vi "SVT Unit Conversion (1 Ch).vi"(0 "spectrum":cluster{"x0":dbl, "dx":dbl, "magnitude":dbl[]} {"magnitude" format="%.2p"; "dx" format="%.2p"; "x0" format="%.2p"}, 1 "desired scaling":T2 {"dB reference (0: no change)" format="%.2f"}, 2 "spectral density desired":T1(ring), 4 "spectrum info in":T3={"channel name"="", "description"="", "x-axis units"=0, "spectral info"={"spectrum type"=enum."Power [Magnitude^2]", "linear/dB"=enum."linear", "window"=0, "window size"=0, "FFT size"=0}, "engineering units"=0, "custom label"="", "dB reference [EU]"=0.0, "peak units"=enum."rms", "weighting filter"=0, "spectral density?"=FALSE, "unit label"="", "spectrum skewed?"=FALSE, "complimentary spectrum units"=enum."none"} {"x-axis units" items=["time"=0, "frequency"=1, "quefrency"=2, "revolutions"=3, "order"=4, "rpm"=11, "rad/s"=21, "index"=65535]; "weighting filter" items=["Linear", "A-weighting", "B-weighting", "C-weighting", "ITU-R 468-4", "Dolby", "CCITT", "C-message"]; "dB reference [EU]" format="%.2f"; "engineering units" items=["custom..."=0, "V"=1, "A"=21, "Pa"=2, "N"=20, "g"=3, "m/s^2"=4, "m/s"=5, "m"=6, "mm/s"=12, "mm"=13, "microns/s"=14, "microns"=15, "in/s^2"=7, "in/s"=8, "in"=9, "mils/s"=10, "mils"=11, "rad/s^2"=16, "rad/s"=17, "rad"=18, "strain"=19]; "spectral info"."window" items=["None "=0, "Hanning"=1, "Hamming"=2, "Blackman-Harris"=3, "Exact Blackman"=4, "Blackman"=5, "Flat Top"=6, "4 Term B-Harris "=7, "7 Term B-Harris"=8, "Low Sidelobe"=9, "Force - Exponential"=10, "Gaussian"=62]}, 5 "error in (no error)":errorcluster) -> (14 "converted spectrum":cluster{"x0":dbl, "dx":dbl, "magnitude":dbl[]} {"magnitude" format="%.2p"; "dx" format="%.2p"; "x0" format="%.2p"}, 15 "unit label":string, 18 "spectrum info out":T3={"channel name"="", "description"="", "x-axis units"=0, "spectral info"={"spectrum type"=enum."Power [Magnitude^2]", "linear/dB"=enum."linear", "window"=0, "window size"=0, "FFT size"=0}, "engineering units"=0, "custom label"="", "dB reference [EU]"=0.0, "peak units"=enum."rms", "weighting filter"=0, "spectral density?"=FALSE, "unit label"="", "spectrum skewed?"=FALSE, "complimentary spectrum units"=enum."none"} {"x-axis units" items=["time"=0, "frequency"=1, "quefrency"=2, "revolutions"=3, "order"=4, "rpm"=11, "rad/s"=21, "index"=65535]; "weighting filter" items=["Linear", "A-weighting", "B-weighting", "C-weighting", "ITU-R 468-4", "Dolby", "CCITT", "C-message"]; "dB reference [EU]" format="%.2f"; "engineering units" items=["custom..."=0, "V"=1, "A"=21, "Pa"=2, "N"=20, "g"=3, "m/s^2"=4, "m/s"=5, "m"=6, "mm/s"=12, "mm"=13, "microns/s"=14, "microns"=15, "in/s^2"=7, "in/s"=8, "in"=9, "mils/s"=10, "mils"=11, "rad/s^2"=16, "rad/s"=17, "rad"=18, "strain"=19]; "spectral info"."window" items=["None "=0, "Hanning"=1, "Hamming"=2, "Blackman-Harris"=3, "Exact Blackman"=4, "Blackman"=5, "Flat Top"=6, "4 Term B-Harris "=7, "7 Term B-Harris"=8, "Low Sidelobe"=9, "Force - Exponential"=10, "Gaussian"=62]}, 19 "error out":errorcluster)   [LabVIEW 2017]
doc: "Converts between dB/linear, Magnitude/Magnitude^2, rms/peak/peak-peak, spectrum/spectral density, and dB ref1/dB ref2. You can use this polymorphic VI to convert a single spectrum, N spectra, a single complex spectrum, N complex spectra, a single channel of XY data, or N channels of XY data. The data type you wire to the <B>spectrum</B> input determines the polymorphic instance to use."
uses:
  <vilib>/addons/Sound and Vibration/compatibility/Controls/svl_Spectrum Info (enhanced).ctl
  <vilib>/addons/Sound and Vibration/compatibility/Controls/svl_Spectrum Type.ctl
  <vilib>/addons/Sound and Vibration/compatibility/Controls/svl_Engineering Units Text Ring.ctl
  <vilib>/addons/Sound and Vibration/compatibility/Controls/svl_Weighting Filter Text Ring.ctl
  <vilib>/addons/Sound and Vibration/compatibility/Controls/svl_Complimentary Spectrum Units.ctl
  <vilib>/addons/_NISVFA/_Spectrum Processing/subVIs/svfa_Peak to RMS to Peak2Peak.vi
  <vilib>/addons/_NISVFA/_Spectrum Processing/subVIs/svfa_Mag to Mag2.vi
  <vilib>/addons/_NISVFA/_Spectrum Processing/subVIs/svfa_Linear to dB.vi
  <vilib>/addons/_NISVFA/_Spectrum Processing/subVIs/svfa_dBrefA to dBrefB.vi
  <vilib>/addons/_NISVFA/_Spectrum Processing/subVIs/svfa_Spectrum to Spectral Density.vi
  <vilib>/addons/_NISVFA/_Shared subVIs/Common/svc_Get Weighting Enum and Labels.vi
  <vilib>/addons/_NISVFA/_Shared subVIs/Common/svc_Unit Label Lexical Class.vi
  <vilib>/addons/_NISVFA/_Shared subVIs/Common/svc_Engineering Units to Unit Label.vi
  <vilib>/addons/_NISVFA/_Shared subVIs/Common/svc_Format Value (DBL).vi
  <vilib>/addons/_NISVFA/_Shared subVIs/Common/svc_Window Parameters.vi
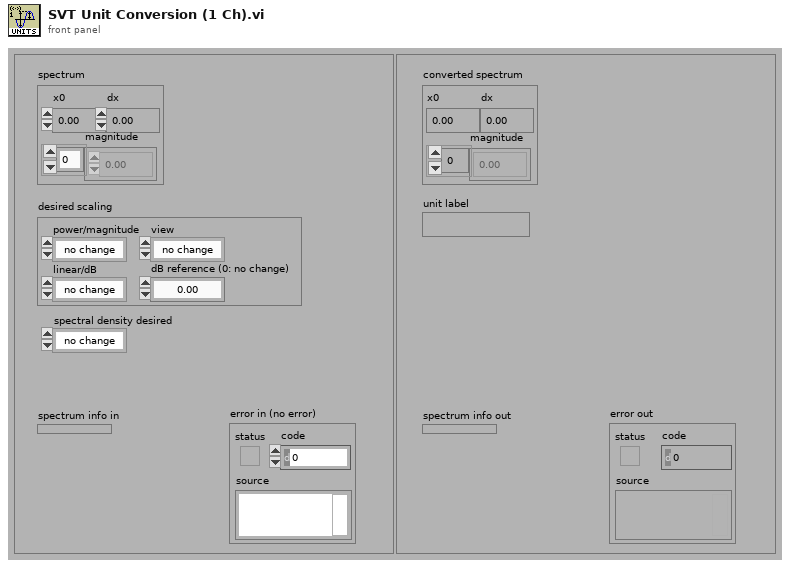
[diagram p1: front panel]
types:
  T1 = enum16{"no change", "spectrum", "spectral density"}
  T2 = cluster{"linear/dB":enum16{"no change", "linear", "dB"}, "dB reference (0: no change)":dbl, "power/magnitude":enum16{"no change", "power", "magnitude"}, "view":enum16{"no change", "rms", "peak", "peak-peak"}}
  T3 = typedef "svl_Spectrum Info (enhanced).ctl" = cluster{"channel name":string, "description":string, "x-axis units":u16, "spectral info":cluster{"spectrum type":T4, "linear/dB":enum16{"linear", "dB"}, "window":u16, "window size":i32, "FFT size":i32}, "engineering units":T5, "custom label":string, "dB reference [EU]":dbl, "peak units":enum16{"rms", "peak", "peak-peak"}, "weighting filter":T6, "spectral density?":bool, "unit label":string, "spectrum skewed?":bool, "complimentary spectrum units":T7}
  T4 = typedef "svl_Spectrum Type.ctl" = enum16{"FFT Spectrum [complex]", "Amplitude [Magnitude]", "Power [Magnitude^2]", "Cross Spectrum [complex]", "Frequency Response [Complex]"}
  T5 = typedef "svl_Engineering Units Text Ring.ctl" = u16
  T6 = typedef "svl_Weighting Filter Text Ring.ctl" = u16
  T7 = typedef "svl_Complimentary Spectrum Units.ctl" = enum16{"none", "radians", "degrees", "cycles", "imaginary"}
  T8 = typedef "svc_Spectrum Info.ctl" = cluster{"channel name":string, "description":string, "x-axis units":T9, "spectral info":cluster{"spectrum type":T10, "linear/dB":enum16{"linear", "dB"}, "window":u16, "window size":i32, "FFT size":i32}, "engineering units":T11, "custom label":string, "dB reference [EU]":dbl, "peak units":enum16{"rms", "peak", "peak-peak"}, "weighting filter":T12, "spectral density?":bool, "unit label":string, "spectrum skewed?":bool, "complimentary spectrum units":T13}
  T9 = typedef "svc_X-Axis Units.ctl" = u16
  T10 = typedef "svc_Spectrum Type.ctl" = enum16{"FFT Spectrum [complex]", "Amplitude [Magnitude]", "Power [Magnitude^2]", "Cross Spectrum [complex]", "Frequency Response [Complex]"}
  T11 = typedef "svc_Engineering Units Text Ring.ctl" = u16
  T12 = typedef "svc_Weighting Filter Text Ring.ctl" = u16
  T13 = typedef "svc_Complimentary Spectrum Units.ctl" = enum16{"none", "radians", "degrees", "cycles", "imaginary"}
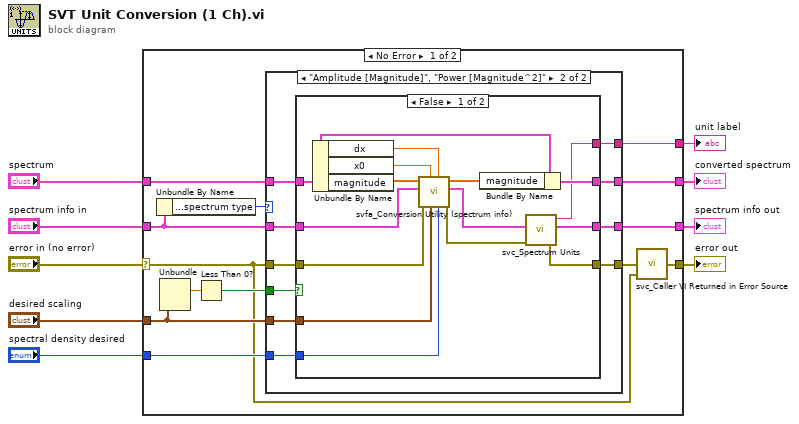
[diagram p0: block diagram]
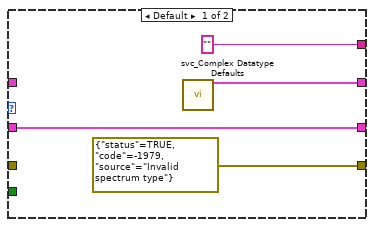
[diagram p2: hidden frame]
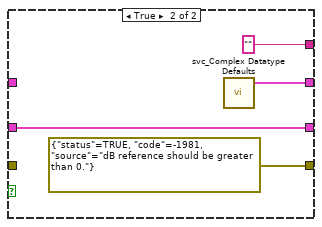
[diagram p3: hidden frame]
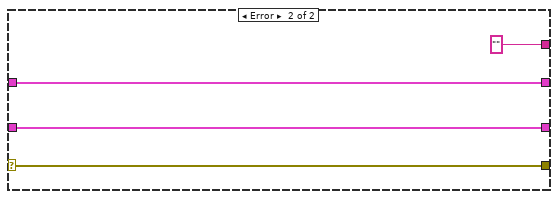
[diagram p4: hidden frame]
diagram:
  n1 = case shown="No Error" "error in (no error)" {
    selector: "error in (no error)" -> [w10 w59]
    tunnel: [w17 w59] -> w8
    tunnel: "spectrum" -> [w22 w56]
    tunnel: "desired scaling" -> [w14 _]
    tunnel: [w21 w56] -> w6
    tunnel: "spectrum info in" -> [w16 w58]
    tunnel: [w18 w58] -> w4
    tunnel: [w19 "" ("unit label")] -> w3
    tunnel: "spectral density desired" -> [w13 _]
    frame No Error {
      n2 = Unbundle By Name(w16) -> ("spectral info.spectrum type"=w15:T4)
      n3 = Unbundle(w14) -> ("dB reference (0: no change)"=w12:dbl)  [unwired: 3 out]
      n4 = Less Than 0?(x=w12) -> (x < 0?=w11:bool)
      n5 = case shown="\"Amplitude [Magnitude]\", \"Power [Magnitude^2]\"" w15 {
        tunnel: w22 -> [_ w36]
        tunnel: [w23 w35] -> w21
        tunnel: w10 -> [_ w34]
        tunnel: w14 -> [_ w33]
        tunnel: [errorcluster {"status"=TRUE, "code"=-1979, "source"="Invalid spectrum type"} ("error out") w32] -> w20
        tunnel: ["" ("unit label") w31] -> w19
        tunnel: [w24 w30] -> w18
        tunnel: w16 -> [w24 w29]
        tunnel: w13 -> [_ w28]
        tunnel: w11 -> [_ w27]
        frame Default {
          n6 = call <vilib>:"svc_Complex Datatype Defaults.vi"() -> ("empty spectrum"=w23:cluster{"f0":dbl, "df":dbl, "magnitude":dbl[]})  [unwired: 11 in, 8 out]
        }
        frame "Amplitude [Magnitude]", "Power [Magnitude^2]" {
          n7 = case shown="False" w27 {
            tunnel: w36 -> [w51 _]
            tunnel: [w50 w52] -> w35
            tunnel: w34 -> [w42 _]
            tunnel: w33 -> [w49 _]
            tunnel: [w47 errorcluster {"status"=TRUE, "code"=-1981, "source"="dB reference should be greater than 0."} ("error out")] -> w32
            tunnel: [w39 "" ("unit label")] -> w31
            tunnel: [w46 w55] -> w30
            tunnel: w29 -> [w43 w55]
            tunnel: w28 -> [w37 _]
            frame False {
              n8 = Unbundle By Name(w51) -> ("dx"=w38:dbl, "x0"=w44:dbl, "magnitude"=w45:dbl[])
              n9 = call <vilib>:"svfa_Conversion Utility (spectrum info).vi"("spectral density desired"=w37, "dx"=w38, "desired scaling"=w49, "x0"=w44, "error in (no error)"=w42, "spectrum info in"=w43, "input signal"=w45) -> ("error out"=w41:errorcluster, "spectrum info out"=w40:T8, "converted signal"=w48:dbl[])  [unwired: 2 in]
              n10 = Bundle By Name(cluster=w51, "magnitude"=w48) -> (w50:cluster{"x0":dbl, "dx":dbl, "magnitude":dbl[]})
              n11 = call <vilib>:"svc_Spectrum Units.vi"("error in (no error)"=w41, "spectrum info in"=w40) -> ("error out"=w47:errorcluster, "spectrum info out"=w46:T8, "unit label"=w39:string)  [unwired: 2 in, 1 out]
            }
            frame True {
              n12 = call <vilib>:"svc_Complex Datatype Defaults.vi"() -> ("empty spectrum"=w52:cluster{"f0":dbl, "df":dbl, "magnitude":dbl[]})  [unwired: 11 in, 8 out]
            }
          }
        }
      }
      n13 = call <vilib>:"svc_Caller VI Returned in Error Source.vi"("warning input to caller"=w10, "error in (no error)"=w20) -> ("error out"=w17:errorcluster)  [unwired: 3 in]
    }
    frame Error {
    }
  }
  "error out" <- w8
  "converted spectrum" <- w6
  "spectrum info out" <- w4
  "unit label" <- w3
